vi "Index Motor Value.vi"(1 "Feed Into Shooter?":dbl) -> (0 "Index Teleop Command":dbl)   [LabVIEW 2019]
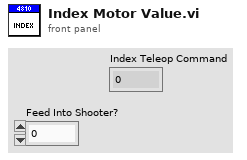
[diagram p1: front panel]
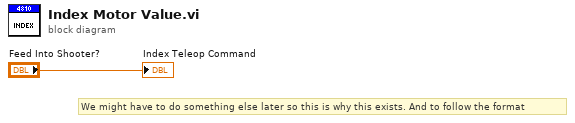
[diagram p0: block diagram]
diagram:
  # "We might have to do something else later so this is why this exists. And to follow the format"
  "Index Teleop Command" <- "Feed Into Shooter?"
